vi "GetWaveform.vi"(8 "error in (no error)":errorcluster caption="错误输入（无错误）", 11 "ChannelTag[]":string[](array[string])) -> (0 "error out":errorcluster caption="错误输出", 1 "Waveform":waveform(dbl)[](array[waveform]), 2 "Valid?":bool)   [LabVIEW 2016]
uses:
  <vilib>/measure/NI_MABase.lvlib
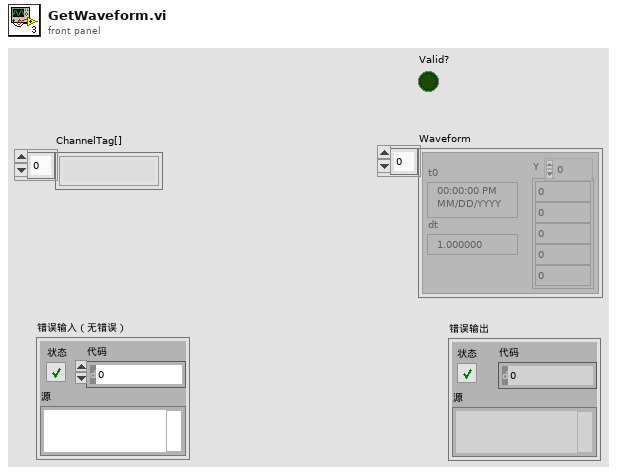
[diagram p1: front panel]
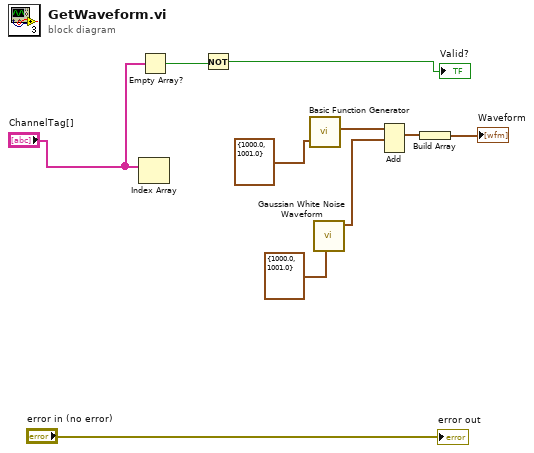
[diagram p0: block diagram]
diagram:
  n1 = Index Array(array="ChannelTag[]") -> ()  [unwired: 1 in, 1 out]
  n2 = Empty Array?(array="ChannelTag[]") -> (empty?=w2:bool)
  n3 = Not(x=w2) -> (.not. x?=→"Valid?":bool)
  n4 = call <vilib>:"Basic Function Generator.vi"("sampling info"=cluster{"Fs":dbl, "#s":dbl} {"Fs"=1000.0, "#s"=1001.0}) -> ("signal out"=w8:waveform(dbl))  [unwired: 8 in, 2 out]
  n5 = call <vilib>:"Gaussian White Noise Waveform.vi"("sampling info"=cluster{"Fs":dbl, "#s":dbl} {"Fs"=1000.0, "#s"=1001.0}) -> ("signal out"=w7:waveform(dbl))  [unwired: 9 in, 1 out]
  n6 = Add(1:w7, 2:w8) -> (0:w5:waveform(dbl))  [unwired: 1 in, 1 out]
  n7 = Build Array(w5) -> (→"Waveform":waveform(dbl)[])
  "error out" <- "error in (no error)"
